vi "String Parsing.vi"() -> ()   [LabVIEW 2019]
panel:
  out "String 4":string="hello world"
  out "String 3":string="hello world"
  out "String 2":string="hello world"
  out "String 1":string="hello world"
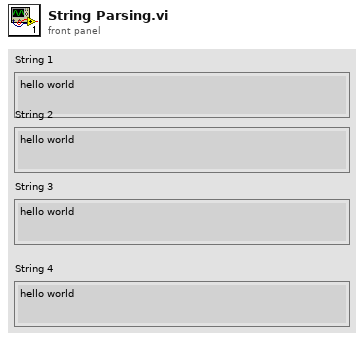
[diagram p1: front panel]
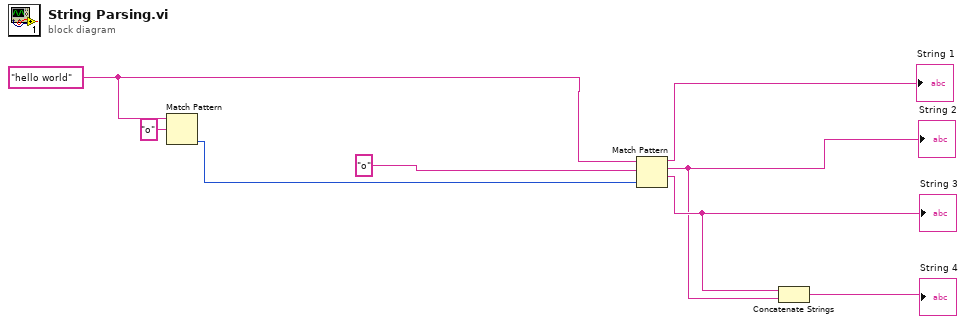
[diagram p0: block diagram]
diagram:
  w3 = "hello world"
  n1 = Match Pattern(string=w3, regular expression="o") -> (offset past match=w1:i32)  [unwired: 1 in, 3 out]
  n2 = Match Pattern(string=w3, regular expression="o", offset (0)=w1) -> (before substring=→"String 1":string, match substring=w5:string, after substring=w6:string)  [unwired: 1 out]
  "String 2" <- w5
  "String 3" <- w6
  n3 = Concatenate Strings(w6, w5) -> (→"String 4":string)
